vi "Generate SysDef Path.vi"() -> (0 "SysDef path":path)   [LabVIEW 2019, in "FPGA Addon Adding Channel Items.lvclass"]
uses:
  FPGA Addon Adding Channel Items.lvclass
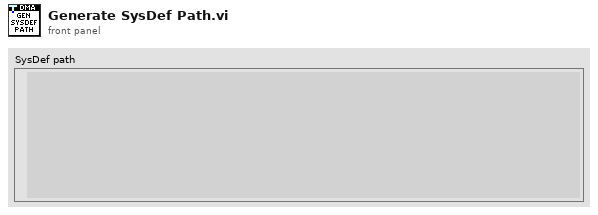
[diagram p1: front panel]
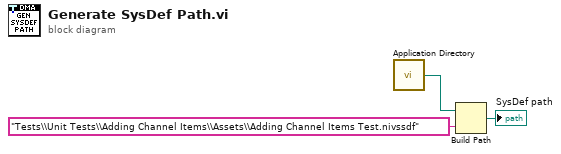
[diagram p0: block diagram]
diagram:
  n1 = call <vilib>:"Application Directory.vi"() -> ("Application Directory"=w3:path)
  n2 = Build Path(base path=w3, name or relative path="Tests\\Unit Tests\\Adding Channel Items\\Assets\\Adding Channel Items Test.nivssdf") -> (appended path=→"SysDef path":path)
